vi "PicoScope6000GetRapidBlockBulk_.vi"(0 "error in":errorcluster, 7 "handle in":i16, 11 "Rapid Block Acquisition Settings":T1={"preTriggerSamples"=0, "postTriggerSamples"=1000, "timebase"=2, "Four Channel Device"=FALSE, "Oversample"=1, "Number of Captures"=1}) -> (2 "Channel A Buffer":i16[][](array[numeric]), 3 "Channel B Buffer":i16[][](array[numeric]), 4 "error out":errorcluster, 6 "handle out":i16, 13 "Channel C Buffer":i16[][](array[numeric]), 14 "Channel D Buffer":i16[][](array[numeric]))   [LabVIEW 2020]
doc: "This VI gets a set of blocks captured using rapid block mode. It outputs two-dimensional arrays for each channel that contain data from all the requested captures."
uses:
  ps6000.dll
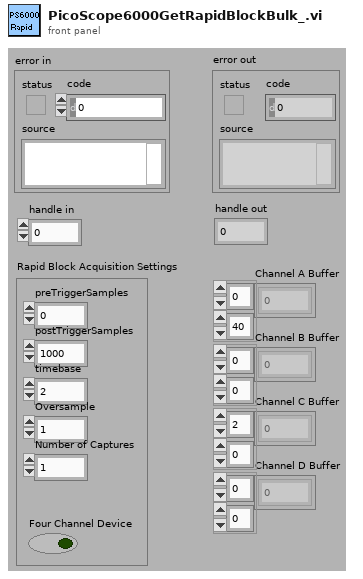
[diagram p1: front panel]
types:
  T1 = cluster{"preTriggerSamples":u32, "postTriggerSamples":u32, "timebase":u32, "Four Channel Device":bool, "Oversample":i16, "Number of Captures":u32}
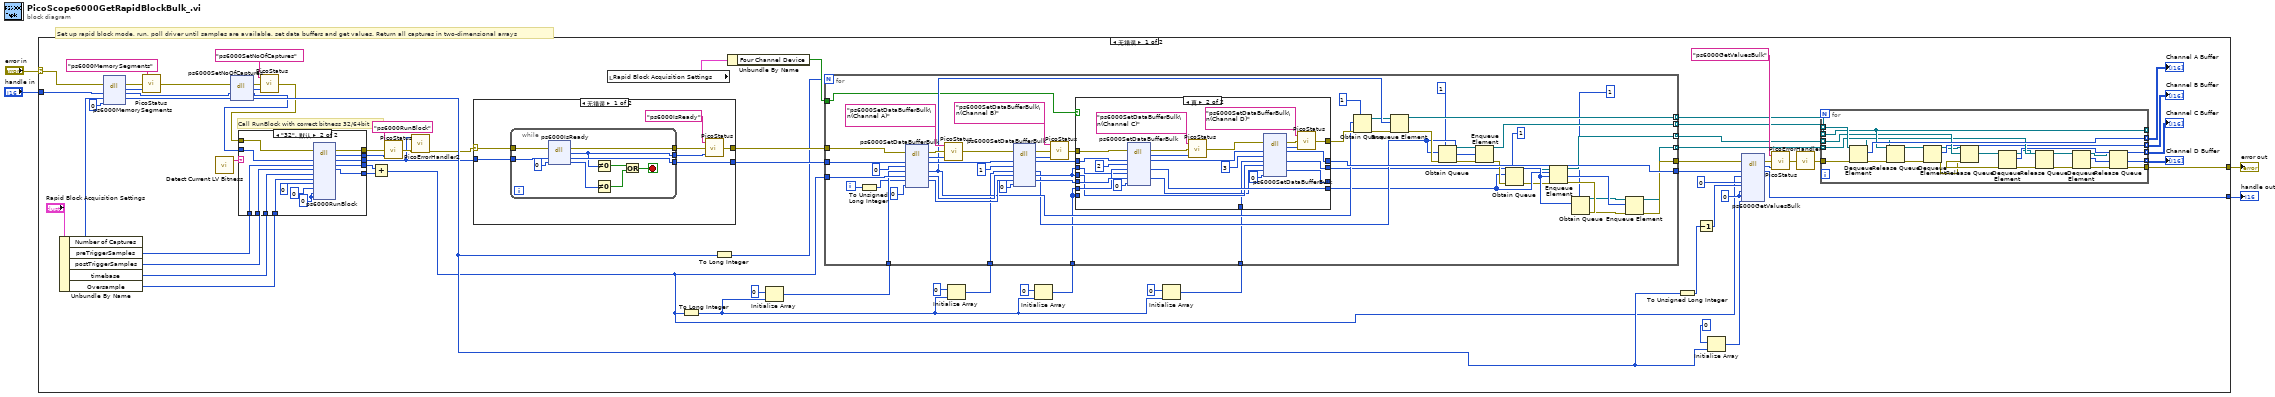
[diagram p0: block diagram]
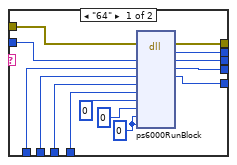
[diagram p2: hidden frame]
diagram:
  # "Set up rapid block mode, run, poll driver until samples are available, set data buffers and get values. Return all captures in two-dimensional arrays"
  n1 = case shown="无错误" "error in" {
    selector: "error in" -> [w68 w226]
    tunnel: [w41 w226] -> w3
    tunnel: "handle in" -> [w67 w225]
    tunnel: [w47 w225] -> w1
    frame No Error {
      w34 = u32 0 ("downSampleRatioMode")
      # "Call RunBlock with correct bitness 32/64bit"
      n2 = Unbundle By Name("Rapid Block Acquisition Settings") -> ("Number of Captures"=w63:u32, "preTriggerSamples"=w8:u32, "postTriggerSamples"=w7:u32, "timebase"=w6:u32, "Oversample"=w5:i16)
      n3 = dll-call lib="PS6000.dll" fn="ps6000MemorySegments" ("ps3000.dll:_ps3000_open_unit@0")(error in=w68, "handle"=w67, "nSegments"=w63, "nMaxSamples"=u32 0) -> (error out=w65:errorcluster, "PICO_STATUS"=w66:u32, "handle"=w61:i16, "nSegments"=w21:u32)  [unwired: 3 in, 1 out]
      n4 = call "PicoStatus.vi"("PICO STATUS"=w66, "error in"=w65, "source"="ps6000MemorySegments") -> ("error out"=w60:errorcluster)
      n5 = call <userlib>:"Detect Current LV Bitness.vi"() -> ("bitness"=w16:string)  [unwired: 11 in]
      n6 = dll-call lib="PS6000.dll" fn="ps6000SetNoOfCaptures" ("ps3000.dll:_ps3000_open_unit@0")(error in=w60, "handle"=w61, "nCaptures"=w21) -> (error out=w58:errorcluster, "PICO_STATUS"=w59:u32, "handle"=w10:i16, "nCaptures"=w22:u32)  [unwired: 2 in, 1 out]
      n7 = call "PicoStatus.vi"("PICO STATUS"=w59, "error in"=w58, "source"="ps6000SetNoOfCaptures") -> ("error out"=w11:errorcluster)
      n8 = case shown="\"32\", 默认" w16 {
        tunnel: w6 -> [w86 w100]
        tunnel: w8 -> [w85 w99]
        tunnel: w7 -> [w84 w98]
        tunnel: [w83 w97] -> w20
        tunnel: [w82 w96] -> w19
        tunnel: w11 -> [w81 w95]
        tunnel: w10 -> [w80 w94]
        tunnel: w5 -> [w79 w93]
        tunnel: [w78 w92] -> w12
        tunnel: [w74 w88] -> w15
        tunnel: [w73 w87] -> w14
        frame "64" {
          w76 = i64 0 ("pParameter")
          n9 = dll-call lib="PS6000.dll" fn="ps6000RunBlock" ("ps3000.dll:_ps3000_open_unit@0")(error in=w81, "handle"=w80, "preTriggerSamples"=w85, "postTriggerSamples"=w84, "timebase"=w86, "oversample"=w79, "timeindisposed"=0 ("pParameter"), "segmentIndex"=i16 0 ("pParameter"), "lpReady"=w76, "pParameter"=w76) -> (error out=w82:errorcluster, "PICO_STATUS"=w83:u32, "handle"=w78:i16, "preTriggerSamples"=w73:u32, "postTriggerSamples"=w74:u32)  [unwired: 8 in, 1 out]
        }
        frame "32", Default {
          w90 = 0 ("pParameter")
          n10 = dll-call lib="PS6000.dll" fn="ps6000RunBlock" ("ps3000.dll:_ps3000_open_unit@0")(error in=w95, "handle"=w94, "preTriggerSamples"=w99, "postTriggerSamples"=w98, "timebase"=w100, "oversample"=w93, "timeindisposed"=0 ("pParameter"), "segmentIndex"=i16 0 ("pParameter"), "lpReady"=w90, "pParameter"=w90) -> (error out=w96:errorcluster, "PICO_STATUS"=w97:u32, "handle"=w92:i16, "preTriggerSamples"=w87:u32, "postTriggerSamples"=w88:u32)  [unwired: 8 in, 1 out]
        }
      }
      n11 = Add(x=w14, y=w15) -> (x+y=w9:u32)
      n12 = call "PicoStatus.vi"("PICO STATUS"=w20, "error in"=w19, "source"="ps6000RunBlock") -> ("error out"=w17:errorcluster)
      n13 = call <userlib>:"PicoErrorHandler2.vi"("error in (no error)"=w17, "handle In"=w12) -> ("error out"=w13:errorcluster)  [unwired: 9 in]
      n14 = case shown="无错误" w13 {
        selector: w13 -> [w210 w223]
        tunnel: w12 -> [w212 w224]
        tunnel: [w211 w224] -> w72
        tunnel: [w209 w223] -> w71
        frame No Error {
          n15 = while {
            tunnel: [w222] -> w211
            tunnel: w212 -> [w221]
            tunnel: [w216] -> w207
            tunnel: w210 -> [w215]
            tunnel: [w214] -> w208
            stop <- w220 stop-if-true
            n16 = dll-call lib="PS6000.dll" fn="ps6000IsReady" ("ps3000.dll:_ps3000_open_unit@0")(error in=w215, "handle"=w221, "ready"=i16 0) -> (error out=w214:errorcluster, "status"=w216:u32, "handle"=w222:i16, "ready"=w217:i16)  [unwired: 2 in, 1 out]
            n17 = Not Equal To 0?(x=w216) -> (x != 0?=w218:bool)
            n18 = Not Equal To 0?(x=w217) -> (x != 0?=w219:bool)
            n19 = Or(x=w218, y=w219) -> (x .or. y?=w220:bool)
          }
          n20 = call "PicoStatus.vi"("PICO STATUS"=w207, "error in"=w208, "source"="ps6000IsReady") -> ("error out"=w209:errorcluster)
        }
        frame Error {
        }
      }
      n21 = local read "Rapid Block Acquisition Settings"() -> (w56:T1)
      n22 = To Long Integer(number=w9) -> (32bit integer=w25:i32)
      n23 = To Long Integer(number=w22) -> (32bit integer=w24:i32)
      n24 = Unbundle By Name(w56) -> ("Four Channel Device"=w69:bool)
      n25 = Initialize Array(i16 0 ("element"), w25) -> (w54:i16[])
      n26 = Initialize Array(i16 0 ("element"), w25) -> (w29:i16[])
      n27 = Initialize Array(i16 0 ("element"), w25) -> (w30:i16[])
      n28 = Initialize Array(i16 0 ("element"), w25) -> (w31:i16[])
      n29 = for {
        N: w24 -> [_]
        tunnel: w72 -> [w175]
        tunnel: w71 -> [w173]
        tunnel: w69 -> [w122]
        tunnel: w9 -> [w167]
        tunnel: w54 -> [w154]
        tunnel: [w153] -> w53
        tunnel: [w145] -> w52
        tunnel: [w143] -> w46 mode=indexing
        tunnel: [w142] -> w45 mode=indexing
        tunnel: [w141] -> w44 mode=indexing
        tunnel: [w140] -> w43 mode=indexing
        tunnel: w31 -> [w127]
        tunnel: w30 -> [w126]
        tunnel: w29 -> [w125]
        i -> [w124]
        n30 = To Unsigned Long Integer(number=w124) -> (unsigned 32bit integer=w123:u32)
        n31 = dll-call lib="PS6000.dll" fn="ps6000SetDataBufferBulk" ("ps3000.dll:_ps3000_open_unit@0")(error in=w173, "handle"=w175, "channel"=0, "buffer"=w154, "bufferLth"=w167, "waveform"=w123, "downSampleRatioMode"=0) -> (error out=w171:errorcluster, "PICO_STATUS"=w172:u32, "handle"=w163:i16, "buffer"=w148:i16[], "bufferLth"=w161:u32, "waveform"=w160:u32)  [unwired: 4 in, 1 out]
        n32 = call "PicoStatus.vi"("PICO STATUS"=w172, "error in"=w171, "source"="ps6000SetDataBufferBulk\n(Channel A)") -> ("error out"=w164:errorcluster)
        n33 = dll-call lib="PS6000.dll" fn="ps6000SetDataBufferBulk" ("ps3000.dll:_ps3000_open_unit@0")(error in=w164, "handle"=w163, "channel"=1, "buffer"=w125, "bufferLth"=w161, "waveform"=w160, "downSampleRatioMode"=0) -> (error out=w166:errorcluster, "PICO_STATUS"=w165:u32, "handle"=w159:i16, "buffer"=w147:i16[], "bufferLth"=w158:u32, "waveform"=w157:u32)  [unwired: 4 in, 1 out]
        n34 = call "PicoStatus.vi"("PICO STATUS"=w165, "error in"=w166, "source"="ps6000SetDataBufferBulk\n(Channel B)") -> ("error out"=w170:errorcluster)
        n35 = case shown="真" w122 {
          tunnel: w159 -> [w178 w196]
          tunnel: [w178 w190] -> w153
          tunnel: w126 -> [w180 w198]
          tunnel: w126 -> [w179 _]
          tunnel: [w179 w192] -> w146
          tunnel: [w180 w200] -> w144
          tunnel: w170 -> [w177 w195]
          tunnel: [w177 w205] -> w152
          tunnel: w158 -> [_ w182]
          tunnel: w158 -> [_ w186]
          tunnel: w157 -> [w176 w199]
          tunnel: [w176 w191] -> _
          tunnel: w127 -> [_ w181]
          frame False {
          }
          frame True {
            n36 = dll-call lib="PS6000.dll" fn="ps6000SetDataBufferBulk" ("ps3000.dll:_ps3000_open_unit@0")(error in=w195, "handle"=w196, "channel"=2, "buffer"=w198, "bufferLth"=w182, "waveform"=w199, "downSampleRatioMode"=0) -> (error out=w202:errorcluster, "PICO_STATUS"=w201:u32, "handle"=w189:i16, "buffer"=w200:i16[], "waveform"=w185:u32)  [unwired: 5 in, 1 out]
            n37 = call "PicoStatus.vi"("PICO STATUS"=w201, "error in"=w202, "source"="ps6000SetDataBufferBulk\n(Channel C)") -> ("error out"=w188:errorcluster)
            n38 = dll-call lib="PS6000.dll" fn="ps6000SetDataBufferBulk" ("ps3000.dll:_ps3000_open_unit@0")(error in=w188, "handle"=w189, "channel"=3, "buffer"=w181, "bufferLth"=w186, "waveform"=w185, "downSampleRatioMode"=0) -> (error out=w194:errorcluster, "PICO_STATUS"=w193:u32, "handle"=w190:i16, "buffer"=w192:i16[], "waveform"=w191:u32)  [unwired: 5 in, 1 out]
            n39 = call "PicoStatus.vi"("PICO STATUS"=w193, "error in"=w194, "source"="ps6000SetDataBufferBulk\n(Channel D)") -> ("error out"=w205:errorcluster)
          }
        }
        n40 = Obtain Queue(max queue size (-1, unlimited)=1, element data type=w148, error in (no error)=w152) -> (queue out=w128:refnum<queue>, error out=w129:errorcluster)  [unwired: 2 in, 1 out]
        n41 = Enqueue Element(queue=w128, element=w148, error in (no error)=w129) -> (queue out=w143:refnum<queue>, error out=w151:errorcluster)  [unwired: 1 in, 1 out]
        n42 = Obtain Queue(max queue size (-1, unlimited)=1, element data type=w147, error in (no error)=w151) -> (queue out=w131:refnum<queue>, error out=w132:errorcluster)  [unwired: 2 in, 1 out]
        n43 = Enqueue Element(queue=w131, element=w147, error in (no error)=w132) -> (queue out=w142:refnum<queue>, error out=w150:errorcluster)  [unwired: 1 in, 1 out]
        n44 = Obtain Queue(max queue size (-1, unlimited)=1, element data type=w144, error in (no error)=w150) -> (queue out=w134:refnum<queue>, error out=w135:errorcluster)  [unwired: 2 in, 1 out]
        n45 = Enqueue Element(queue=w134, element=w144, error in (no error)=w135) -> (queue out=w141:refnum<queue>, error out=w149:errorcluster)  [unwired: 1 in, 1 out]
        n46 = Obtain Queue(max queue size (-1, unlimited)=1, element data type=w146, error in (no error)=w149) -> (queue out=w137:refnum<queue>, error out=w138:errorcluster)  [unwired: 2 in, 1 out]
        n47 = Enqueue Element(queue=w137, element=w146, error in (no error)=w138) -> (queue out=w140:refnum<queue>, error out=w145:errorcluster)  [unwired: 1 in, 1 out]
      }
      n48 = To Unsigned Long Integer(number=w22) -> (unsigned 32bit integer=w23:u32)
      n49 = Decrement(x=w23) -> (x-1=w36:u32)
      n50 = Initialize Array(i16 0, w22) -> (w35:i16[])
      n51 = dll-call lib="PS6000.dll" fn="ps6000GetValuesBulk" ("ps3000.dll:_ps3000_open_unit@0")(error in=w52, "handle"=w53, "NoOfsamples"=w9, "FromSegmentIndex"=u32 0, "ToSegmentIndex"=w36, "DownSampleRatio"=w34, "downSampleRatioMode"=w34, "overflow"=w35) -> (error out=w50:errorcluster, "PICO_STATUS"=w49:u32, "handle"=w47:i16)  [unwired: 8 in, 1 out]
      n52 = call "PicoStatus.vi"("PICO STATUS"=w49, "error in"=w50, "source"="ps6000GetValuesBulk") -> ("error out"=w48:errorcluster)
      n53 = call <userlib>:"PicoErrorHandler.vi"("error in"=w48) -> ("error out"=w40:errorcluster)
      n54 = for {
        tunnel: w46 -> [w121] mode=indexing
        tunnel: [w114] -> _ mode=indexing
        tunnel: w45 -> [w114] mode=indexing
        tunnel: w44 -> [w113] mode=indexing
        tunnel: w43 -> [w112] mode=indexing
        tunnel: [w120] -> w42 mode=indexing
        tunnel: [w118] -> w41
        tunnel: w40 -> [w115]
        tunnel: [w111] -> w39 mode=indexing
        tunnel: [w110] -> w38 mode=indexing
        tunnel: [w109] -> w37 mode=indexing
        n55 = Dequeue Element(queue=w121, error in (no error)=w115) -> (queue out=w102:refnum<queue>, element=w120:i16[], error out=w101:errorcluster)  [unwired: 1 in, 1 out]
        n56 = Release Queue(queue=w102, error in (no error)=w101) -> (error out=w116:errorcluster)  [unwired: 1 in, 2 out]
        n57 = Dequeue Element(queue=w114, error in (no error)=w116) -> (queue out=w104:refnum<queue>, element=w109:i16[], error out=w103:errorcluster)  [unwired: 1 in, 1 out]
        n58 = Release Queue(queue=w104, error in (no error)=w103) -> (error out=w117:errorcluster)  [unwired: 1 in, 2 out]
        n59 = Dequeue Element(queue=w113, error in (no error)=w117) -> (queue out=w106:refnum<queue>, element=w110:i16[], error out=w105:errorcluster)  [unwired: 1 in, 1 out]
        n60 = Release Queue(queue=w106, error in (no error)=w105) -> (error out=w119:errorcluster)  [unwired: 1 in, 2 out]
        n61 = Dequeue Element(queue=w112, error in (no error)=w119) -> (queue out=w108:refnum<queue>, element=w111:i16[], error out=w107:errorcluster)  [unwired: 1 in, 1 out]
        n62 = Release Queue(queue=w108, error in (no error)=w107) -> (error out=w118:errorcluster)  [unwired: 1 in, 2 out]
      }
      "Channel D Buffer" <- w39
      "Channel C Buffer" <- w38
      "Channel B Buffer" <- w37
      "Channel A Buffer" <- w42
    }
    frame Error {
    }
  }
  "error out" <- w3
  "handle out" <- w1
